vi "FestoCPX.Station.TowerLed.Fglb.vi"(7 "Action (get)":T2=enum."get", 8 "error in":errorcluster, 10 "Blink period [ms]":u32, 11 "Color":T1) -> (0 "error out":errorcluster, 1 "Trigger":bool, 2 "Color out":T1)   [LabVIEW 2016]
uses:
  FestoCPX.Station.TowerLed.Fglb.Action.ctl
  FestoCPX.Station.TowerLed.Color.ctl
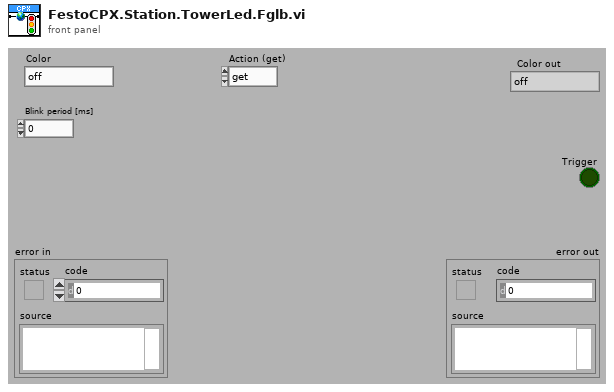
[diagram p1: front panel]
types:
  T1 = typedef "FestoCPX.Station.TowerLed.Color.ctl" = enum16{"off", "red", "orange", "green", "green/orange"}
  T2 = typedef "FestoCPX.Station.TowerLed.Fglb.Action.ctl" = enum16{"init", "set", "get"}
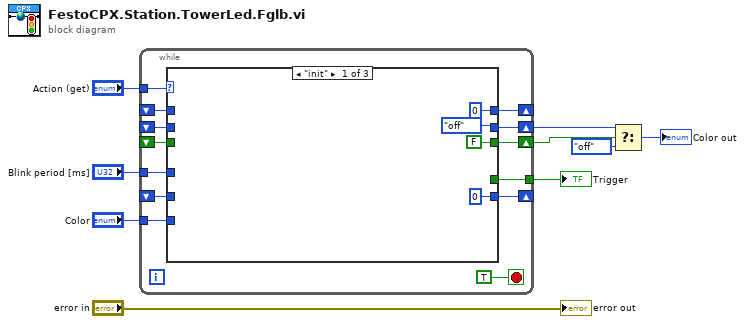
[diagram p0: block diagram]
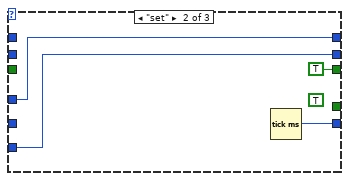
[diagram p2: hidden frame]
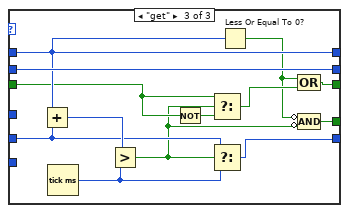
[diagram p3: hidden frame]
diagram:
  n1 = while {
    tunnel: "Action (get)" -> [w21]
    tunnel: "Blink period [ms]" -> [w20]
    shift-right: [w19] -> _
    shift-left: _ -> [w18]
    tunnel: "Color" -> [w17]
    shift-right: [w15] -> w3
    shift-left: _ -> [w16]
    shift-right: [w14] -> w4
    shift-left: _ -> [w13]
    shift-right: [w12] -> _
    shift-left: _ -> [w11]
    tunnel: [w10] -> w5
    stop <- TRUE stop-if-true
    n2 = case shown="\"init\"" w21 {
      tunnel: w20 -> [_ w28 _]
      tunnel: [u32 0 ("millisecond timer value") w27 w39] -> w19
      tunnel: w18 -> [_ _ w41]
      tunnel: w17 -> [_ w30 _]
      tunnel: [FALSE TRUE w37] -> w15
      tunnel: w16 -> [_ _ w36]
      tunnel: [FestoCPX.Station.TowerLed.Color."off" ("Color") w30 w43] -> w14
      tunnel: w13 -> [_ _ w43]
      tunnel: [u32 0 ("Blink period [ms]") w28 w38] -> w12
      tunnel: w11 -> [_ _ w38]
      tunnel: [_ _ w31] -> w10
      frame "init" {
      }
      frame "set" {
        (unwired) TRUE
        n3 = Tick Count (ms)() -> (millisecond timer value=w27:u32)
      }
      frame "get" {
        n4 = Add(x=w38, y=w41) -> (x+y=w42:u32)
        n5 = Tick Count (ms)() -> (millisecond timer value=w40:u32)
        n6 = Greater?(x=w42, y=w40) -> (0:w32:bool)
        n7 = Not(x=w36) -> (.not. x?=w35:bool)
        n8 = Select(t=w36, s=w32, f=w35) -> (s? t:f=w34:bool)
        n9 = Select(t=w41, s=w32, f=w40) -> (s? t:f=w39:u32)
        n10 = Less Or Equal To 0?(x=w38) -> (x <= 0?=w33:bool)
        n11 = Compound Arithmetic op=OR(w33, w34) -> (w37:bool)
        n12 = Compound Arithmetic op=AND(invert w33, invert w32) -> (w31:bool)
      }
    }
  }
  "Trigger" <- w5
  n13 = Select(t=w4, s=w3, f=FestoCPX.Station.TowerLed.Color."off") -> (s? t:f=→"Color out":T1)
  "error out" <- "error in"
